vi "Login Request.vi"(8 "error in (no error)":errorcluster, 9 "password":string, 10 "username":string, 11 "[P] User in":refnum<class "[P] User.lvclass">) -> (0 "error out":errorcluster, 3 "[P] User out":refnum<class "[P] User.lvclass">)   [LabVIEW 2020, in "[P] User.lvlib" / "[P] User.lvclass"]
uses:
  [P] User.lvclass
  [V] Login/[V] Login Messages/Login Fail Msg/Login Fail Msg.lvclass
  <vilib>/ActorFramework/Stop Msg/Stop Msg.lvclass
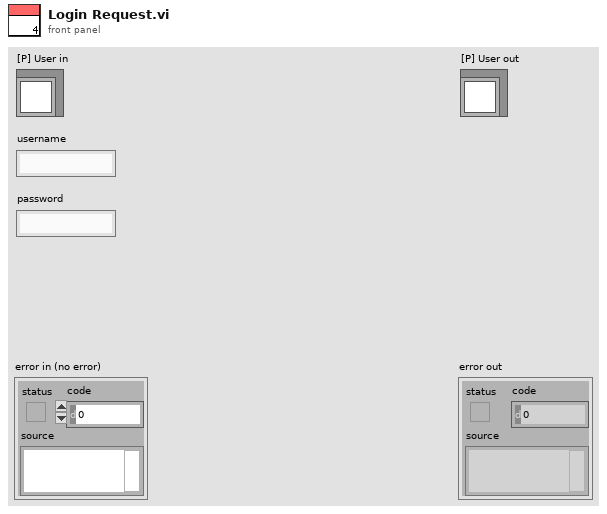
[diagram p1: front panel]
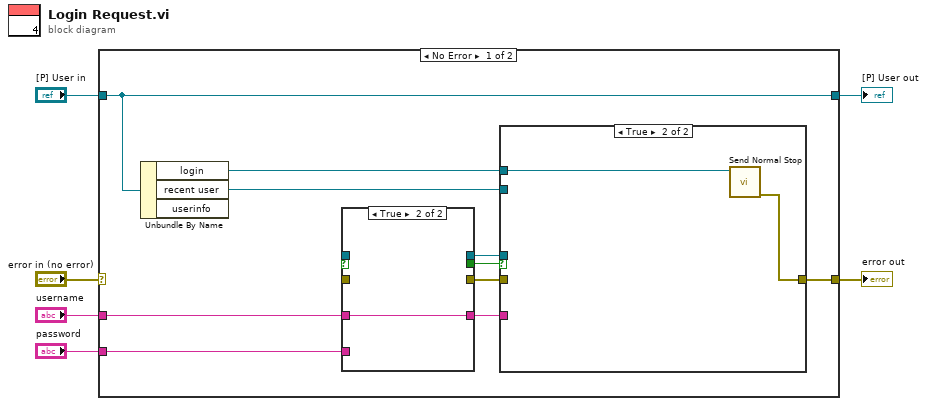
[diagram p0: block diagram]
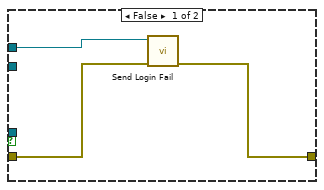
[diagram p2: hidden frame]
diagram:
  n1 = case shown="No Error" "error in (no error)" {
    selector: "error in (no error)" -> [w21 w44]
    tunnel: [w11 w44] -> w3
    tunnel: "[P] User in" -> [w8 w43]
    tunnel: [w8 w43] -> w4
    tunnel: "username" -> [w15 _]
    tunnel: "password" -> [w16 _]
    frame No Error {
      n2 = Unbundle By Name(w8) -> ("login"=w9:refnum<class "Message Enqueuer.lvclass">, "recent user"=w7:refnum<class "[Data] Recent User.lvclass">, "userinfo"=w20:refnum<class "[Data] Abstruct Userinfo.lvclass">)
      n3 = case shown="True" w18 {
        selector: [w33 _] -> w18
        tunnel: [w34 w41] -> w19
        tunnel: [w35 w42] -> w17
        tunnel: [w35 w39] -> w12
        tunnel: [w34 w38] -> w14
        tunnel: w16 -> [_ w40]
        tunnel: w15 -> [w32 w36]
        tunnel: [w33 w37] -> w13
        tunnel: [w32 w36] -> w10
        frame False {
        }
        frame True {
        }
      }
      n4 = case shown="True" w13 {
        tunnel: w14 -> [w24 w31]
        tunnel: w12 -> [_ w30]
        tunnel: [w22 w28] -> w11
        tunnel: w10 -> [_ w25]
        tunnel: w9 -> [w23 w29]
        tunnel: w7 -> [_ w27]
        frame False {
          n5 = call "Send Login Fail.vi"("error in (no error)"=w24, "Message Enqueuer"=w23) -> ("error out"=w22:errorcluster)  [unwired: 8 in, 1 out]
        }
        frame True {
          n6 = call <vilib>:"Send Normal Stop.vi"("Message Enqueuer"=w29) -> ("error out"=w28:errorcluster, "error in (no error)"=w26:errorcluster)  [unwired: 9 in]
        }
      }
    }
    frame Error {
    }
  }
  "error out" <- w3
  "[P] User out" <- w4
